vi "ZYNQMsg_Identifier.vi"(10 "Enable":bool, 11 "Message":string) -> ()   [LabVIEW 2014]
uses:
  c_MicroZedMsg.ctl
  g_MicroZed_Interface.vi
  g_ReportControl.vi
  g_ChipData.vi
panel:
  out "element":bool
  in  "Combo Box":T1
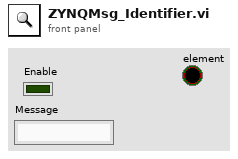
[diagram p1: front panel]
types:
  T1 = typedef "c_MicroZedMsg.ctl" = string
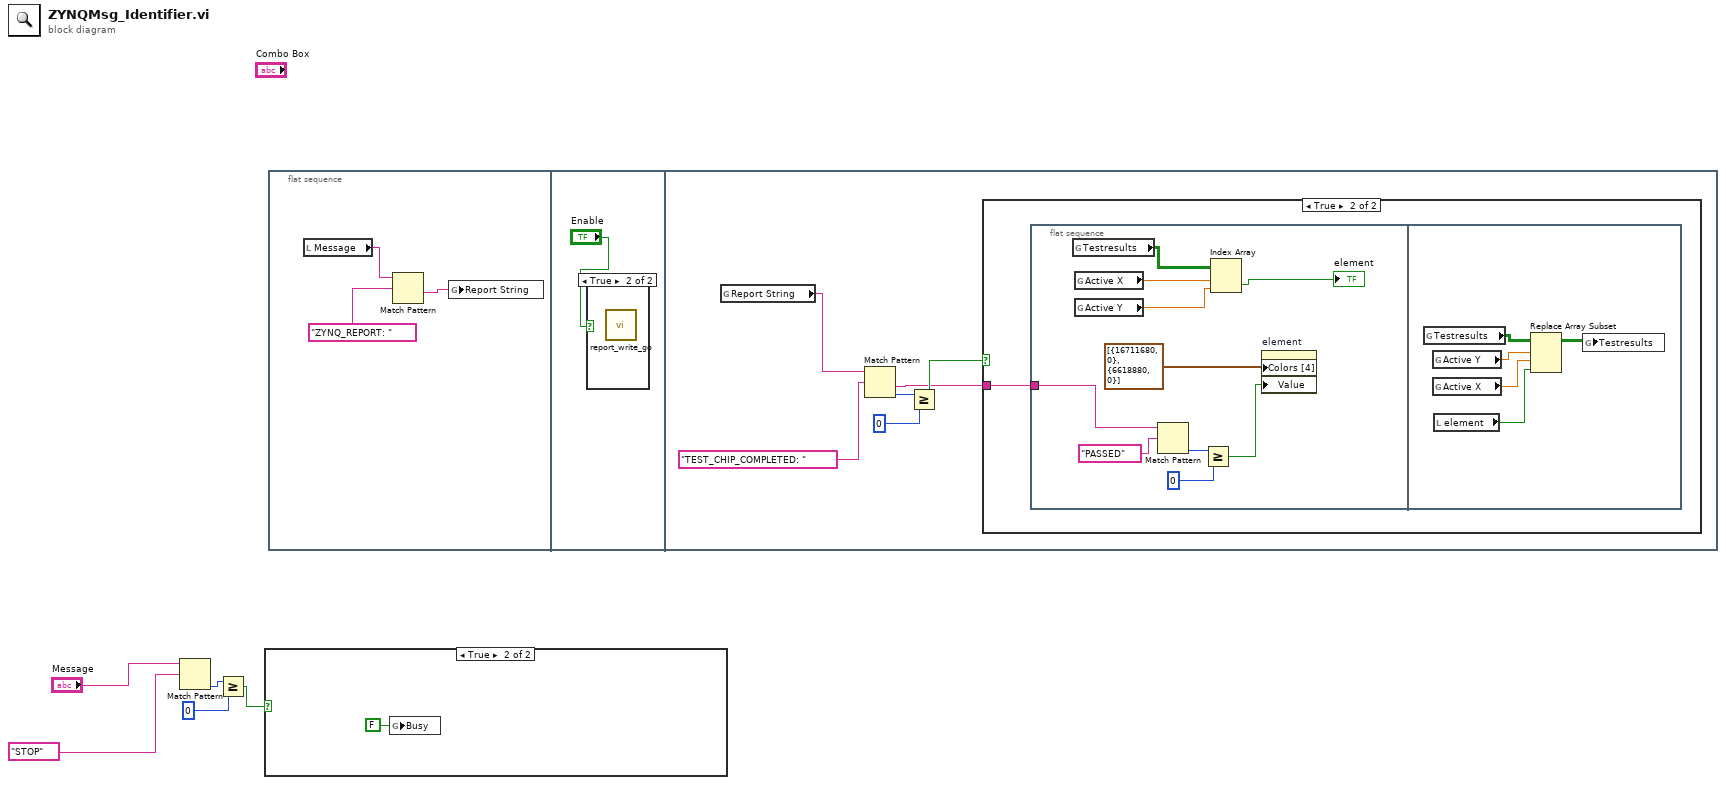
[diagram p0: block diagram]
diagram:
  n1 = Match Pattern(string="Message", regular expression=T1 "STOP" ("Combo Box")) -> (offset past match=w4:i32)  [unwired: 1 in, 3 out]
  n2 = Greater Or Equal?(x=w4, y=0) -> (x >= y?=w2:bool)
  n3 = case shown="True" w2 {
    frame False {
    }
    frame True {
      n4 = global write "g_MicroZed_Interface.vi" "Busy"(FALSE ("Busy")) -> ()
    }
  }
  n5 = flat-sequence {
    frame #0 {
      n6 = local read "Message"() -> (w8:string)
      n7 = Match Pattern(string=w8, regular expression=T1 "ZYNQ_REPORT: " ("Combo Box")) -> (after substring=w7:string)  [unwired: 1 in, 3 out]
      n8 = global write "g_ReportControl.vi" "Report String"(w7) -> ()
    }
    frame #1 {
      n9 = case shown="True" "Enable" {
        frame False {
        }
        frame True {
          n10 = call "report_write_go.vi"() -> ()  [unwired: 12 in]
        }
      }
    }
    frame #2 {
      n11 = global read "g_ReportControl.vi" "Report String"() -> (w11:string)
      n12 = Match Pattern(string=w11, regular expression=T1 "TEST_CHIP_COMPLETED: " ("Combo Box")) -> (after substring=w13:string, offset past match=w16:i32)  [unwired: 1 in, 2 out]
      n13 = Greater Or Equal?(x=w16, y=0) -> (x >= y?=w14:bool)
      n14 = case shown="True" w14 {
        tunnel: w13 -> [_ w17]
        frame False {
        }
        frame True {
          n15 = flat-sequence {
            tunnel: w17 -> [w22]
            frame #0 {
              n16 = global read "g_ChipData.vi" "Testresults"() -> (w27:bool[][])
              n17 = global read "g_ChipData.vi" "Active X"() -> (w26:dbl)
              n18 = global read "g_ChipData.vi" "Active Y"() -> (w25:dbl)
              n19 = Match Pattern(string=w22, regular expression=T1 "PASSED" ("Combo Box")) -> (offset past match=w19:i32)  [unwired: 1 in, 3 out]
              n20 = Greater Or Equal?(x=w19, y=0) -> (x >= y?=w18:bool)
              n21 = Index Array(array=w27, index (row)=w26, index (col)=w25) -> (element=→"element":bool)
              n22 = property on="element" class="Bool (strict)"("Colors [4]"=cluster{u32, u32}[] [{16711680, 0}, {6618880, 0}], "Value"=w18) -> ()  [unwired: 2 in, 2 out]
            }
            frame #1 {
              n23 = global read "g_ChipData.vi" "Testresults"() -> (w32:bool[][])
              n24 = global read "g_ChipData.vi" "Active Y"() -> (w31:dbl)
              n25 = global read "g_ChipData.vi" "Active X"() -> (w30:dbl)
              n26 = local read "element"() -> (w29:bool)
              n27 = Replace Array Subset(array=w32, new element=w29, index (row)=w31, index (col)=w30) -> (w28:bool[][])
              n28 = global write "g_ChipData.vi" "Testresults"(w28) -> ()
            }
          }
        }
      }
    }
  }
